vi "CH1_accumutator_V.vi"(11 "Vin":dbl) -> (3 "voltage_acc":dbl)   [LabVIEW 2012]
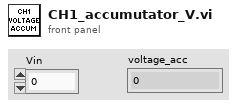
[diagram p1: front panel]
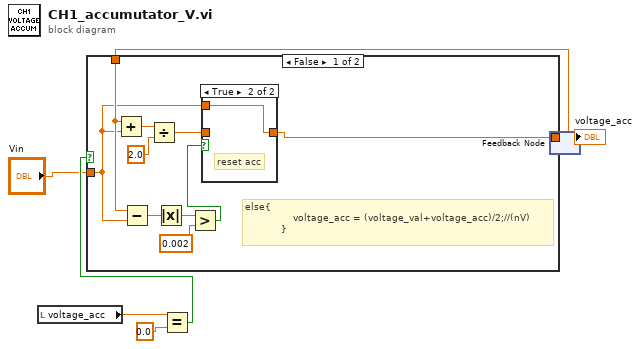
[diagram p0: block diagram]
diagram:
  n1 = local read "voltage_acc"() -> (w4:dbl)
  n2 = Equal?(x=w4, y=0.0) -> (x = y?=w5:bool)
  n3 = feedback #1() -> (w1:dbl)  [unwired: 1 in]
  "voltage_acc" <- w1
  n4 = case shown="False" w5 {
    tunnel: "Vin" -> [w7 w19]
    tunnel: [w9 w19] -> w2
    tunnel: w1 -> [w8 _]
    frame False {
      # "else{\n                voltage_acc = (voltage_val+voltage_acc)/2;//(nV)\n            }"
      n5 = Add(x=w8, y=w7) -> (x+y=w16:dbl)
      n6 = Subtract(x=w8, y=w7) -> (x-y=w10:dbl)
      n7 = Divide(x=w16, y=2.0) -> (x/y=w12:dbl)
      n8 = Absolute Value(x=w10) -> (abs(x)=w11:dbl)
      n9 = Greater?(x=w11, y=0.002) -> (0:w13:bool)
      n10 = case shown="True" w13 {
        tunnel: w12 -> [w17 _]
        tunnel: [w17 w18] -> w9
        tunnel: w7 -> [_ w18]
        frame False {
        }
        frame True {
          # "reset acc"
        }
      }
    }
    frame True {
      # "if(voltage_acc == 0){\n    voltage_acc = voltage_val;\n}"
    }
  }
  n11 = feedback-in #1(w2) -> ()
